vi "LCSS classification brute force.vi"(8 "length match match (60)":dbl=60.0 format="%#_13g", 9 "Percentage match (80)":dbl=80.0 format="%#_13g", 10 "Include zero transitions (t)":bool=TRUE, 11 "Full transition sequence from service to end":string[](array[string])=["-2 0 3 0 -3 0 4 -4 0\r\n", "0 3\r\n", "0 4 -3 0 -4 1 0 4 -3 0\r\n", "0\r\n", "-2 0 3 -3 0 -4 1 -4 0 3 -3 4 -3 0 2 0 3\r\n", "0 3 0 1\r\n", "0 1 0 3\r\n", "0 3 -2 0 4\r\n", "0\r\n", "0 -3 4 0 2 -2 0 -3 0 3 -2 3 -3 4\r\n", "0 -3 4 -3 0\r\n", "-2 0 -2 2 0\r\n", "0 3 -2\r\n", "0 4 -3 0 3 -2 0 -3 4 -3 0 3 -2 2 -2 0 4 0\r\n", "2 0 1 -4 0 3 0 -4 4 0 -4 4 0 2 0 4 0 -3 4 -3 0 -4 0 4\r\n", "0 4\r\n", "-2 0 -2 0 3 0\r\n", "0 3 0 -2 3\r\n", "0 4 0 4 -4 0 2 0 -4 4 -3 0 -2 2 -2 0 4 -3 0 2 0 3 0\r\n", "0 4 -3 0 1 -1 0 3 0 -2 2 -2 0 -3 4 -3 0 4 -4 1 0\r\n", "", "0 -3\r\n", "2 0 3 0 1 0 -2 3\r\n", "0\r\n", "1 -1 0\r\n", "0 -2 3 0\r\n", "0 1 0 4 0 4 -4 4\r\n", "0 1 -1 0 3\r\n", "0 2 -2 3 -3 4\r\n", "-2 2 0 -2 3\r\n", "0 -1\r\n", "0 4 -4 4 0 3 0 -2 0 -4 0 1 -4\r\n", "-2 0 4 0 -3 3 0 -2 2 -2 0 -4 0 4 0\r\n", "0 -1 0 -4 4 -4 1 -4 0\r\n", "1 -4 1 0 2 0 -3 0 2 0 -2 0 1 0 1 -4 4 -4 1 0 3 -2 0 -4 4 -4\r\n", "0 1 -4 4 -4 1\r\n", "0 3 0 -3 3 0 1 0 1 -4 4\r\n", "0 1 -4 0 1 -4\r\n", "0 3 -2 0 1 -4 1 0 2 0 4 0 4 0 -1 2 -1 0\r\n", "1 0 -1 0 2 0 4 -4\r\n", "-4\r\n", "-1 0 4\r\n", "0 1 -1 0 1 -4 0\r\n", "-1 0 1 -4 0 3 0 2 0 4 0 -4 4 -4 0 -1 0 -4 0 -2 0 4\r\n", "0 4 0\r\n", "0 4 -4 0 2 -1 0 2 0 4 -4 1 -4 4 0 3\r\n", "0 4 0 2 0\r\n", "1 0 -1 1 0 -4 1 -4 1 0 -4\r\n", "0 3 -2 0 -4\r\n", "2 -1 0 -4 4 -4 0 2 0 4\r\n", "1 0\r\n", "-1 0 -1 1 0 -4\r\n", "0 3 0\r\n", "0 -4 4 -4 0 -4 0 4 0 2 0 1 -4 4\r\n", "-1 0 1 -4\r\n", "-1 0 2 -1 0 2\r\n", "1 -1 0 4 -4 1\r\n", "-1 0 1 -4 4 -4 0 -4 4\r\n", "0 3 0 3 0 1 -1 0 1\r\n", "-1 0 4 0 4 -4 1 0 -4 0\r\n", "1 0 4\r\n", "0 -1 0 2 -1 0 -2 3 -2 0 -4 4 -4\r\n", "0 3 0\r\n", "2 -1 0 1 -4 4 -4 0 2 0\r\n", "0 4 -4 1 0 1 0 1 -4 0 2 0 4 0 4 -4 1\r\n", "1 -1 0 3 0 3 0 1 0 4\r\n", "0 -4 0 -2 0 -4\r\n", "0 -4 4 -4 0 -2 0 2 0\r\n", "-1 0 4 -4 0\r\n", "1 0 -1 2 0 4\r\n", "0 2 0 -2 0\r\n", "0 1 -4 0 -4 0 3 -2 0 -4 0 -4 4 -4 1\r\n", "0 4 0 4 0 4 0 4 0 -2 3 0 3 0 4 0\r\n", "-4 -1\r\n", "-2 0 1 0 -4 4\r\n", "0 4\r\n", "-2 2 0 -1 -4 1 0 3 0\r\n", "-1 0 -1 2\r\n", "0 -1 1 0 4 0 3 -2 0 -2 3 -2 0 4 0 -2 2\r\n", "2 -1 0 4\r\n", "0 4 0 2 0 -2 0\r\n", "1 -1 0 3 0 -4 4 -4 0\r\n", "2 -1 0 3 -2 0 -3 0 3 0 -3 0\r\n", "0 4 0 4 -4 1 -1 0 -3 0 1 -4 1 0 4 0 -4 0 -4 4 -4 1\r\n", "0 -4 1 0 -4 4\r\n", "0 4 0 -2 2 -2 2 -2 2\r\n", "-2 2 -1 0 4 0 2 0 4 0 2 -2 0 4\r\n", "1 0 -1 0 -1 0 1 -1\r\n", "-2 2 -2 3\r\n", "1 0 -1 0 -1 2 0 2 -2 0 -4 0\r\n", "-2 2 0 3 -2 2\r\n", "0\r\n", "1 -1 0 3\r\n", "0 4 0\r\n", "-2 0 1 -4 0 -3 0\r\n", "1 0 -1 2 -1 1 -4\r\n", "0 4\r\n", "-2 0 -1 1\r\n", "0 3 0 3 0 3 -2\r\n", "-4 0 -4 4\r\n", "0 4 0 -4 0 -4\r\n", "-2 2 0 4 -4 0 2 -2\r\n", "-2 2 -2 0 -1\r\n", "0 4 -3 0\r\n", "0 1 0 -1 1\r\n", "-4 0\r\n", "-2 0 3 0 1 0 3 -2 0 -1 0 4 0 3 0 -3 3 -3\r\n", "0 4 0 -2 0 1 0 -4 4 -3 0 1 0 4 0 -4 1 0 3 -3 0\r\n", "0 -1 2\r\n", "2 0 -3 4 0\r\n", "-4 0 -3 3 -3 0 -3 3 0 -2 3 0\r\n", "0 -1 1 -4 4 -3 0 3 0\r\n", "0 -1 2 0 3 0 1 -4 4 0 2 0\r\n", "2 -2 0 -4 0 -4 4 0 -4\r\n", "1 -1 2 -1\r\n", "2 0 -2 0 4 0 2 0 3 0 -2 0 -4\r\n", "1 -1 0 -1\r\n", "0 1 -4 1\r\n", "0 4 0 -1 1 -1 0\r\n", "0 3\r\n", "-2 0\r\n", "1 -4 0 -2 0 4 0 -4 0 4 -3 0 1 -4 0 1\r\n", "0 -3 3 -2 0 3 0 -2 2\r\n", "1 0\r\n", "2\r\n", "0 -4\r\n", "0 4 0 -4 0 -3 3 -3 0 -2 0 -2 0 4 0 -1 1 0 3 0 -4 1 -4 0 4\r\n", "2 0 -1 1\r\n", "0 2 0 4 0 4 -4 0 -1 2\r\n", "0 3 -2 0 3 -2\r\n", "1 0 -3 3 0 -4\r\n", "0 -3 3 0 -1 0\r\n", "2 -2 0 1\r\n", "-4 1 -4 1 -4 0\r\n", "0 4 0 2 0 -4 1 2 -1 0 4 0 1 0 4 -4 4 0 -4 4 0\r\n", "-2 0 3 0 -2 0\r\n"]) -> (2 "Output (Highest LCSS match, Pattern being matched, matching patterns)":string[][](array[string]))   [LabVIEW 2013]
panel:
  out "LCSS match percentage":i32[][](array[numeric])
  out "LCSS value array":string[][](array[string])
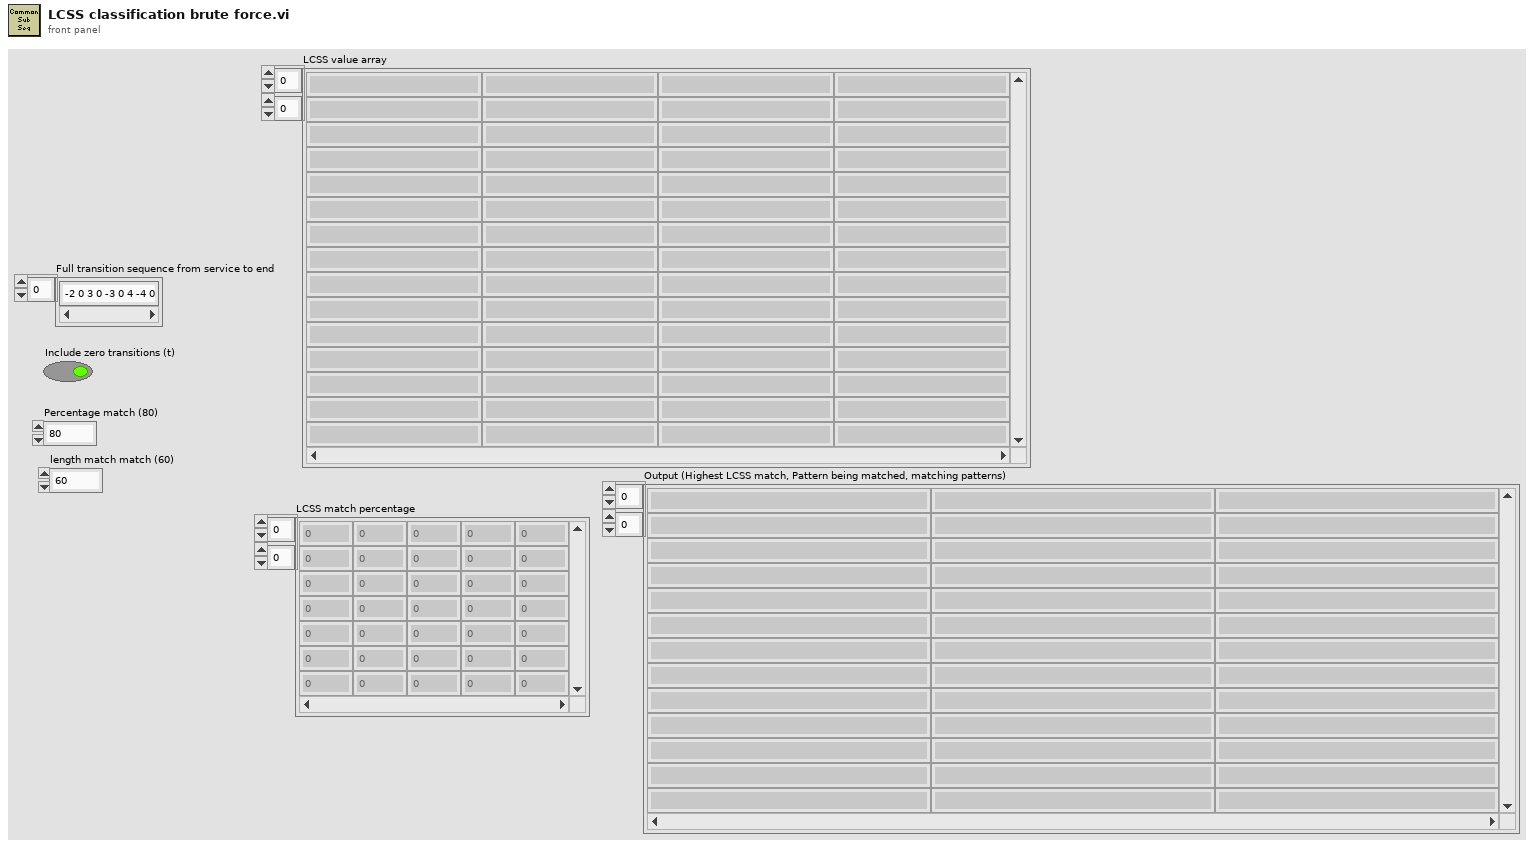
[diagram p1: front panel]
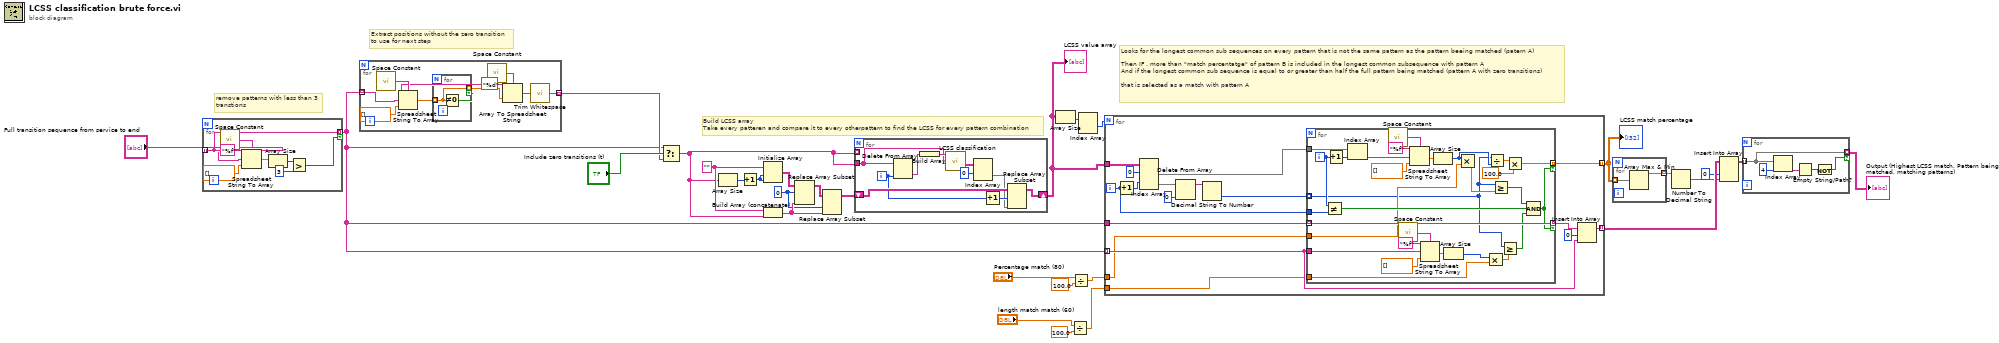
[diagram p0: block diagram]
diagram:
  w23 = 0 ("index (row)")
  w27 = ""
  # "Looks for the longest common sub sequences on every pattern that is not the same pattern as the pattern beeing matched (patern A)\n\nThen IF , more than \"match percentatge\" of pattern B is included in the longest common subsequence with pattern A\nAnd if the longest common sub sequence is equal to or greater than half the full pattern being matched (pattern A with zero transitions)\n \nthat is selected as a match with pattern A"
  # "Build LCSS array\nTake every patteren and compare it to every otherpattern to find the LCSS for every pattern combination"
  # "Extract positions without the zero transition\nto use for next step"
  # "remove patterns with less than 3\ntranstions"
  n1 = for {
    tunnel: "Full transition sequence from service to end" -> [w31] mode=indexing
    tunnel: [w31] -> w8 mode=indexing if=w30
    n2 = call <vilib>:"Space Constant.vi"() -> ("String"=w36:string)
    n3 = Spreadsheet String To Array(delimiter (Tab)=w36, format string="%f", spreadsheet string=w31, array type (2D Dbl)=dbl[] [] ("array 2")) -> (array=w34:dbl[])
    n4 = Array Size(array=w34) -> (size(s)=w33:i32)
    n5 = Greater?(x=w33, y=3) -> (0:w30:bool)
  }
  n6 = for {
    tunnel: w8 -> [w44] mode=indexing
    tunnel: [w38] -> w9 mode=indexing
    w41 = "%d" ("format string")
    n7 = call <vilib>:"Space Constant.vi"() -> ("String"=w46:string)
    n8 = Spreadsheet String To Array(delimiter (Tab)=w46, format string=w41, spreadsheet string=w44, array type (2D Dbl)=dbl[] [] ("array 2")) -> (array=w43:dbl[])
    n9 = for {
      tunnel: w43 -> [w48] mode=indexing
      tunnel: [w48] -> w42 mode=indexing if=w47
      n10 = Not Equal To 0?(x=w48) -> (x != 0?=w47:bool)
    }
    n11 = call <vilib>:"Space Constant.vi"() -> ("String"=w40:string)
    n12 = Array To Spreadsheet String(delimiter (Tab)=w40, array=w42, 3:w41) -> (spreadsheet string=w39:string)
    n13 = call <vilib>:"Trim Whitespace.vi"("string"=w39) -> ("trimmed string"=w38:string)  [unwired: 1 in]
  }
  n14 = Select(t=w8, s="Include zero transitions (t)", f=w9) -> (s? t:f=w10:string[])
  n15 = Array Size(array=w10) -> (size(s)=w29:i32)
  n16 = Increment(x=w29) -> (x+1=w28:i32)
  n17 = Initialize Array(w27, w28, w28) -> (w26:string[][])
  n18 = Build Array (concatenate)(w27, w10) -> (w24:string[])
  n19 = Replace Array Subset(array=w26, new element=w24, index (row)=w23) -> (w25:string[][])  [unwired: 1 in]
  n20 = Replace Array Subset(array=w25, new element=w24, index (col)=w23) -> (w22:string[][])  [unwired: 1 in]
  n21 = for {
    tunnel: w10 -> [_] mode=indexing
    tunnel: w10 -> [w49]
    shift-right: [w53] -> w16
    shift-left: w22 -> [w56]
    i -> [w54]
    n22 = Delete From Array(array=w49, index=w54) -> (deleted portion=w58:string)  [unwired: 1 in, 1 out]
    n23 = Build Array(w58) -> (w57:string[])
    n24 = call "LCSS classification.vi"("cluster centers"=w49, "Patterns in"=w57) -> ("patterns in, distance values"=w52:string[][])  [unwired: 7 in, 2 out]
    n25 = Index Array(array=w52, index (row)=0) -> (element=w50:string[])  [unwired: 1 in]
    n26 = Increment(x=w54) -> (x+1=w55:i32)
    n27 = Replace Array Subset(array=w56, new element=w50, index (row)=w55) -> (w53:string[][])  [unwired: 1 in]
  }
  "LCSS value array" <- w16
  n28 = Array Size(array=w16) -> (size(s)=w21:i32[])
  n29 = Divide(x="length match match (60)", y=100.0) -> (x/y=w2:dbl)
  n30 = Divide(x="Percentage match (80)", y=100.0) -> (x/y=w5:dbl)
  n31 = Index Array(array=w21) -> (element #1=w14:i32)  [unwired: 2 in, 1 out]
  n32 = for {
    N: w14 -> [_]
    tunnel: w16 -> [w75]
    tunnel: [w67] -> w20 mode=indexing
    tunnel: [w64] -> w13 mode=indexing
    tunnel: w8 -> [w63]
    tunnel: w8 -> [w61] mode=indexing
    tunnel: w5 -> [w60]
    tunnel: w2 -> [w59]
    i -> [w66]
    n33 = Increment(x=w66) -> (x+1=w62:i32)
    n34 = Index Array(array=w75, index (row) #1=0 ("index (row)"), index (row) #2=w62) -> (element #1=w69:string[], element #2=w71:string[])  [unwired: 2 in]
    n35 = Delete From Array(array=w71, index=0) -> (array with subset deleted=w73:string[])  [unwired: 1 in, 1 out]
    n36 = Decimal String To Number(string=w73) -> (number=w72:i32[])  [unwired: 2 in, 1 out]
    n37 = for {
      tunnel: w72 -> [w79] mode=indexing
      tunnel: [w94] -> w64 mode=indexing if=w81
      tunnel: [w87] -> w65 mode=indexing if=w81
      tunnel: w69 -> [w104]
      tunnel: w66 -> [w102]
      tunnel: w63 -> [w87] mode=indexing
      tunnel: w61 -> [w85]
      tunnel: w60 -> [w80]
      tunnel: w59 -> [w76]
      i -> [w103]
      n38 = Not Equal?(x=w103, y=w102) -> (x != y?=w82:bool)
      n39 = Increment(x=w103) -> (x+1=w93:i32)
      n40 = Index Array(array=w104, index=w93) -> (element=w92:string)
      n41 = call <vilib>:"Space Constant.vi"() -> ("String"=w100:string)
      n42 = call <vilib>:"Space Constant.vi"() -> ("String"=w90:string)
      n43 = Spreadsheet String To Array(delimiter (Tab)=w100, format string="%f", spreadsheet string=w92, array type (2D Dbl)=dbl[] [] ("array 2")) -> (array=w98:dbl[])
      n44 = Spreadsheet String To Array(delimiter (Tab)=w90, format string="%f", spreadsheet string=w85, array type (2D Dbl)=dbl[] [] ("array 2")) -> (array=w88:dbl[])
      n45 = Array Size(array=w98) -> (size(s)=w86:i32)
      n46 = Array Size(array=w88) -> (size(s)=w77:i32)
      n47 = Multiply(x=w86, y=w80) -> (x*y=w97:dbl)
      n48 = Multiply(x=w77, y=w76) -> (x*y=w78:dbl)
      n49 = Divide(x=w79, y=w86) -> (x/y=w96:dbl)
      n50 = Greater Or Equal?(x=w79, y=w97) -> (x >= y?=w84:bool)
      n51 = Greater Or Equal?(x=w79, y=w78) -> (x >= y?=w83:bool)
      n52 = Multiply(x=w96, y=100.0) -> (x*y=w94:dbl)
      n53 = Compound Arithmetic op=AND(w84, w82, w83) -> (w81:bool)
    }
    n54 = Insert Into Array(array=w65, index=0, new element=w61) -> (w67:string[])
  }
  "LCSS match percentage" <- w13
  n55 = for {
    tunnel: w13 -> [w106] mode=indexing
    tunnel: [w105] -> w12 mode=indexing
    n56 = Array Max & Min(array=w106) -> (max value=w105:dbl)  [unwired: 3 out]
  }
  n57 = Number To Decimal String(number=w12) -> (decimal integer string=w19:string[])  [unwired: 1 in]
  n58 = Insert Into Array(array=w20, index (col)=0 ("disabled index (col)"), new element=w19) -> (w17:string[][])  [unwired: 1 in]
  n59 = for {
    tunnel: w17 -> [w108] mode=indexing
    tunnel: [w108] -> w15 mode=indexing if=w107
    n60 = Index Array(array=w108, index=4) -> (element=w110:string)
    n61 = Empty String/Path?(string/path=w110) -> (empty?=w109:bool)
    n62 = Not(x=w109) -> (.not. x?=w107:bool)
  }
  "Output (Highest LCSS match, Pattern being matched, matching patterns)" <- w15
